vi "Hessian ij element.vi"(1 "Fn":u16(ring) items=["Error", "Test"], 2 "d rel":dbl[](array[numeric])=[10.0, 1.0, 0.0, 0.1, 1.0, 1.0, 1.0, 1.0, 1.0, 1.0] format="%_4g", 3 "d":dbl=0.0010000000000000002 format="%_4g", 4 "j":dbl, 5 "i":dbl, 6 "Array":dbl[](array[numeric])=[7.0, 0.61, 0.5, 1.522, 0.11, 0.36, 0.5, 0.24, 0.055, 1.0] format="%_4g") -> (0 "Hij":dbl)   [LabVIEW 2016]
panel:
  out "Array 2":dbl[][](array[numeric])
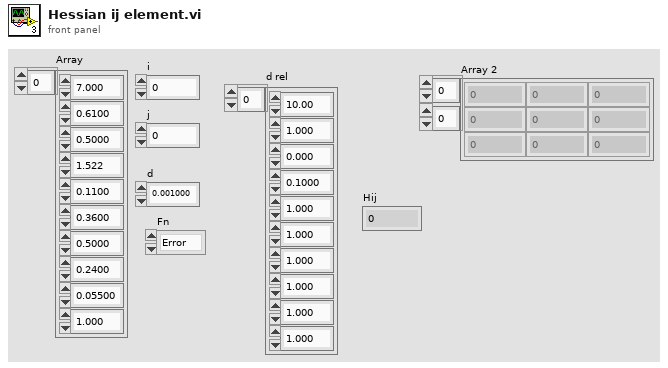
[diagram p1: front panel]
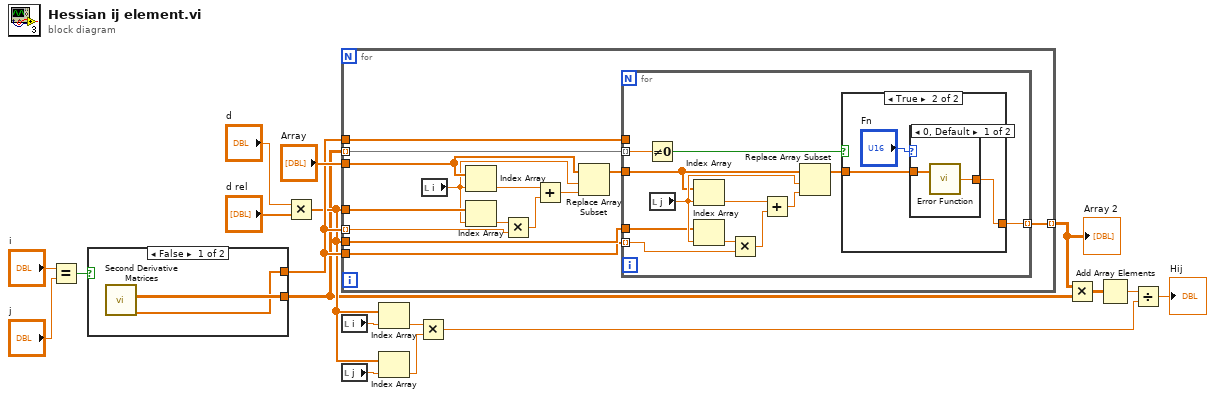
[diagram p0: block diagram]
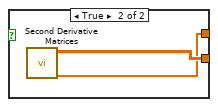
[diagram p2: hidden frame]
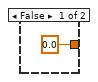
[diagram p3: hidden frame]
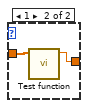
[diagram p4: hidden frame]
diagram:
  n1 = Equal?(x="i", y="j") -> (x = y?=w16:bool)
  n2 = case shown="False" w16 {
    tunnel: [w20 w22] -> w2
    tunnel: [w19 w21] -> w12
    frame False {
      n3 = call "Second Derivative Matrices.vi"() -> ("d2/dxdy"=w20:dbl[][], "d"=w19:dbl[])  [unwired: 2 in, 2 out]
    }
    frame True {
      n4 = call "Second Derivative Matrices.vi"() -> ("d2/dx2"=w22:dbl[][], "d"=w21:dbl[])  [unwired: 2 in, 2 out]
    }
  }
  n5 = Multiply(x="d", y="d rel") -> (x*y=w10:dbl[])
  n6 = for {
    tunnel: w12 -> [w35]
    tunnel: w2 -> [w36] mode=indexing
    tunnel: "Array" -> [w34]
    tunnel: w12 -> [w31] mode=indexing
    tunnel: w10 -> [w30]
    tunnel: w10 -> [w26]
    tunnel: w12 -> [w24]
    tunnel: [w23] -> w3 mode=indexing
    n7 = local read "i"() -> (w29:dbl)
    n8 = Index Array(array=w34, index=w29) -> (element=w33:dbl)
    n9 = Index Array(array=w30, index=w29) -> (element=w25:dbl)
    n10 = Multiply(x=w25, y=w31) -> (x*y=w32:dbl)
    n11 = Add(x=w33, y=w32) -> (x+y=w28:dbl)
    n12 = Replace Array Subset(array=w34, new element=w28, index=w29) -> (w27:dbl[])
    n13 = for {
      tunnel: w36 -> [w47] mode=indexing
      tunnel: w27 -> [w43]
      tunnel: w35 -> [_]
      tunnel: w26 -> [w41]
      tunnel: w24 -> [w39] mode=indexing
      tunnel: [w37] -> w23 mode=indexing
      n14 = Not Equal To 0?(x=w47) -> (x != 0?=w48:bool)
      n15 = local read "j"() -> (w45:dbl)
      n16 = Index Array(array=w43, index=w45) -> (element=w44:dbl)
      n17 = Index Array(array=w41, index=w45) -> (element=w40:dbl)
      n18 = Multiply(x=w40, y=w39) -> (x*y=w38:dbl)
      n19 = Add(x=w44, y=w38) -> (x+y=w46:dbl)
      n20 = Replace Array Subset(array=w43, new element=w46, index=w45) -> (w42:dbl[])
      n21 = case shown="True" w48 {
        tunnel: [0.0 ("Error") w52] -> w37
        tunnel: w42 -> [_ w51]
        frame False {
        }
        frame True {
          n22 = case shown="0, Default" "Fn" {
            tunnel: [w54 w55] -> w52
            tunnel: w51 -> [w53 w56]
            frame 0, Default {
              n23 = call "Error Function.vi"("Array"=w53) -> ("Error"=w54:dbl)  [unwired: 1 in]
            }
            frame 1 {
              n24 = call "Test function.vi"("Array"=w56) -> ("Error"=w55:dbl)  [unwired: 10 in]
            }
          }
        }
      }
    }
  }
  "Array 2" <- w3
  n25 = local read "i"() -> (w11:dbl)
  n26 = local read "j"() -> (w9:dbl)
  n27 = Index Array(array=w10, index=w11) -> (element=w7:dbl)
  n28 = Index Array(array=w10, index=w9) -> (element=w8:dbl)
  n29 = Multiply(x=w7, y=w8) -> (x*y=w5:dbl)
  n30 = Multiply(x=w3, y=w2) -> (x*y=w1:dbl[][])
  n31 = Add Array Elements(numeric array=w1) -> (sum=w6:dbl)
  n32 = Divide(x=w6, y=w5) -> (x/y=→"Hij":dbl)
